vi "ni579x Initialize EEPROM (5792).vi"(0 "Register Bus":refnum<class "ni579x Register Bus v1 Host.lvclass">=refnum, 1 "scope":string(combo)="characterization data eeprom", 5 "start address":u32 format="%x", 11 "Error In":errorcluster) -> (4 "Register Bus (out)":refnum<class "ni579x Register Bus v1 Host.lvclass">, 15 "Error Out":errorcluster)   [LabVIEW 2015]
uses:
  <instrlib>/ni579x/Register Bus/v1/Host/ni579x Register Bus v1 Host.lvclass
  <instrlib>/ni579x/Config/v1/Shared/Types/EEPROM/ni579x EEPROM Header.ctl
  <instrlib>/ni579x/Config/v1/Shared/Types/EEPROM/ni579x EEPROM Calibration Header.ctl
  <instrlib>/ni579x/Config/v1/Shared/Types/EEPROM/ni579x EEPROM Device Data Header.ctl
panel:
  in  "Device Data Header":T1={"Checksum"=0, "Number of Channels"=1, "Number of Attenuations"=[255], "Number of Attenuator Settings"=[2], "Number of Gain Settings"=[64], "Pointer to Cal Data"=[160], "Number of Reserved Bytes"=7, "Number of Frequencies"=[168]} {"Checksum" format="%x"}
  in  "EEPROM Calibration Header":T2={"Checksum"=0, "Date"=timestamp(0 s since 1904-01-01), "Temperature"=25.0, "Misc. Info"="", "Pointer to Device Data Header"=128, "Number of Reserved Bytes"=28} {"Checksum" format="%x"}
  in  "EEPROM Header":T3={"Checksum"=0, "Product Code"=30299, "Hardware Current Version"=1, "Hardware Oldest Compatible Version"=1, "EEPROM Map Current Version"=0, "EEPROM Map Oldest Compatible Version"=0, "User Password"="", "Pointer to Factory Header"=64, "Pointer to User Header"=0, "Recommended Interval"=12, "Number of Reserved Bytes"=32} {"Product Code" format="%x"; "Checksum" format="%x"}
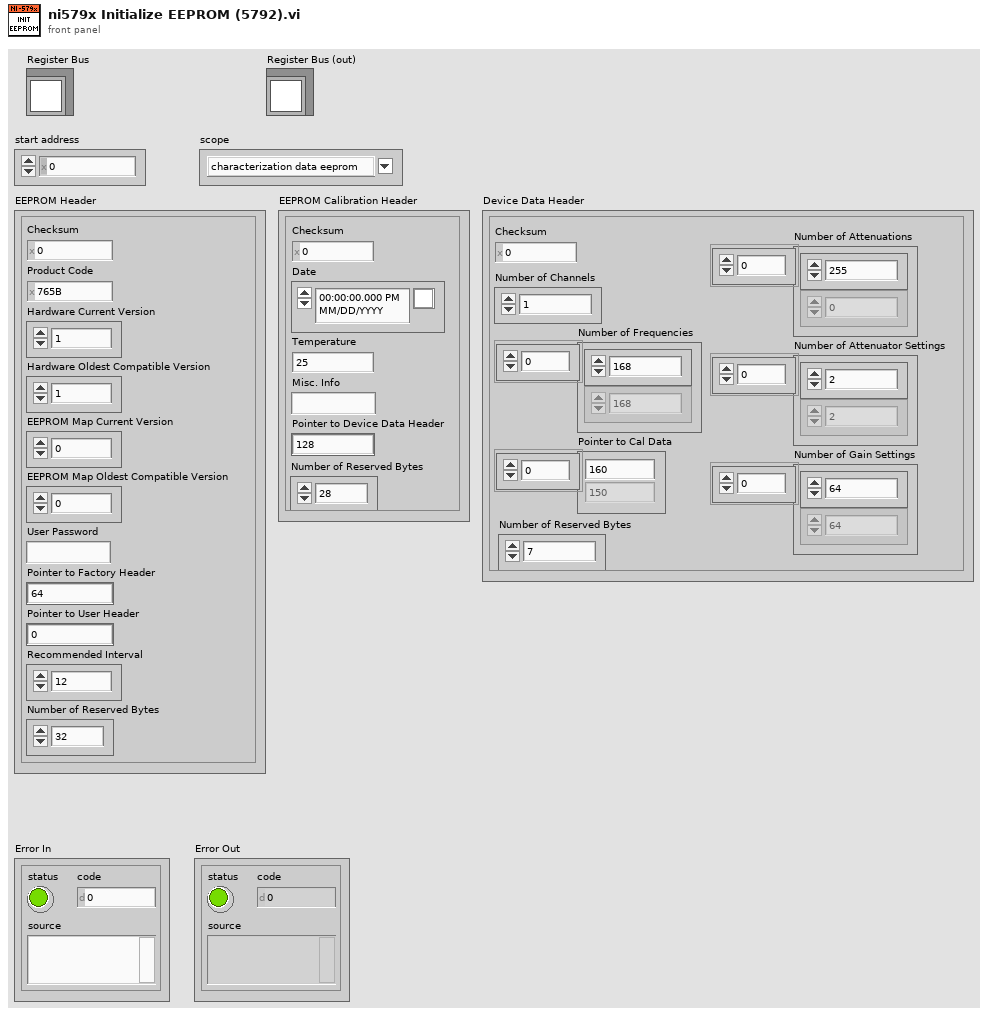
[diagram p1: front panel]
types:
  T1 = typedef "ni579x EEPROM Device Data Header.ctl" = cluster{"Checksum":u32, "Number of Channels":u8, "Number of Attenuations":u16[], "Number of Attenuator Settings":u8[], "Number of Gain Settings":u8[], "Pointer to Cal Data":u32[], "Number of Reserved Bytes":i32, "Number of Frequencies":u16[]}
  T2 = typedef "ni579x EEPROM Calibration Header.ctl" = cluster{"Checksum":u32, "Date":timestamp, "Temperature":sgl, "Misc. Info":string, "Pointer to Device Data Header":u32, "Number of Reserved Bytes":i32}
  T3 = typedef "ni579x EEPROM Header.ctl" = cluster{"Checksum":u32, "Product Code":u16, "Hardware Current Version":u16, "Hardware Oldest Compatible Version":u16, "EEPROM Map Current Version":u16, "EEPROM Map Oldest Compatible Version":u16, "User Password":string, "Pointer to Factory Header":u32, "Pointer to User Header":u32, "Recommended Interval":u16, "Number of Reserved Bytes":i32}
  T4 = typedef "ni579x Characterization Data.ctl" = cluster{"Attenuation Table [dB]":dbl[][], "Frequencies [Hz]":dbl[], "IQ Imbalance Table":T5[], "Gain Table":T6[][]}
  T5 = typedef "ni579x IQ Imbalance.ctl" = cluster{"Gain Imbalance [linear]":dbl, "Phase Imbalance [radians]":dbl, "Offset":cdb}
  T6 = typedef "ni579x Gain to Attenuation Mapping.ctl" = cluster{"Actual Gain [dB]":dbl, "Attenuation Table Index":i32}
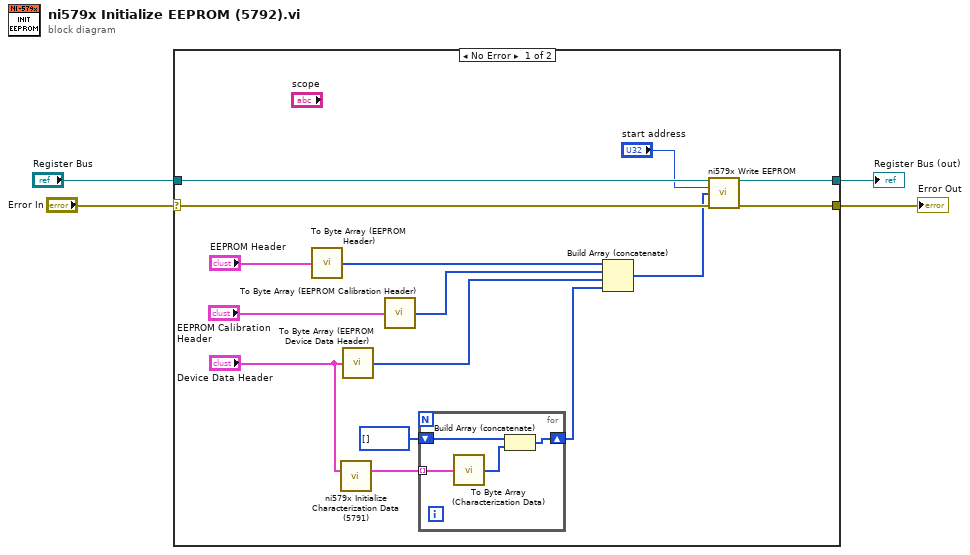
[diagram p0: block diagram]
diagram:
  n1 = case shown="No Error" "Error In" {
    selector: "Error In" -> [w17 w25]
    tunnel: [w16 w25] -> w3
    tunnel: "Register Bus" -> [w19 w24]
    tunnel: [w18 w24] -> w1
    frame No Error {
      n2 = call <instrlib>:"To Byte Array (EEPROM Header).vi"("EEPROM Header"="EEPROM Header") -> ("byte array out"=w12:u8[])
      n3 = call <instrlib>:"ni579x Initialize Characterization Data (5791).vi"("Device Data Header"="Device Data Header") -> ("Characterization Data"=w8:T4[])  [unwired: 13 in, 1 out]
      n4 = call <instrlib>:"To Byte Array (EEPROM Device Data Header).vi"("Device Data Header"="Device Data Header") -> ("byte array out"=w10:u8[])
      n5 = call <instrlib>:"To Byte Array (EEPROM Calibration Header).vi"("EEPROM Calibration Header"="EEPROM Calibration Header") -> ("byte array out"=w11:u8[])
      n6 = for {
        tunnel: w8 -> [w23] mode=indexing
        shift-right: [w21] -> w6
        shift-left: u8[] [] -> [w20]
        n7 = call <instrlib>:"To Byte Array (Characterization Data).vi"("Characterization Data"=w23) -> ("byte array out"=w22:u8[])
        n8 = Build Array (concatenate)(w20, w22) -> (w21:u8[])
      }
      n9 = Build Array (concatenate)(w12, w11, w10, w6) -> (w5:u8[])
      n10 = call <instrlib>:"ni579x Write EEPROM.vi"("Register Bus"=w19, "start address"="start address", "data"=w5, "Error In"=w17) -> ("Register Bus (out)"=w18:refnum<class "ni579x Register Bus v1 Host.lvclass">, "Error Out"=w16:errorcluster)  [unwired: 10 in]
    }
    frame Error {
    }
  }
  "Register Bus (out)" <- w1
  "Error Out" <- w3
